vi "update-signal-values.vi"(8 "error in (no error)":errorcluster, 9 "Array":bool[](array[boolean]), 10 "TAGS":string[](array[string]), 11 "dbc in":refnum<class "dbc.lvclass">) -> (0 "error out":errorcluster, 3 "dbc out":refnum<class "dbc.lvclass">)   [LabVIEW 2015, in "dbc.lvclass"]
uses:
  dbc.lvclass
  dbc.lvclass/dbc.ctl
  <resource>/objmgr/xnet.rc
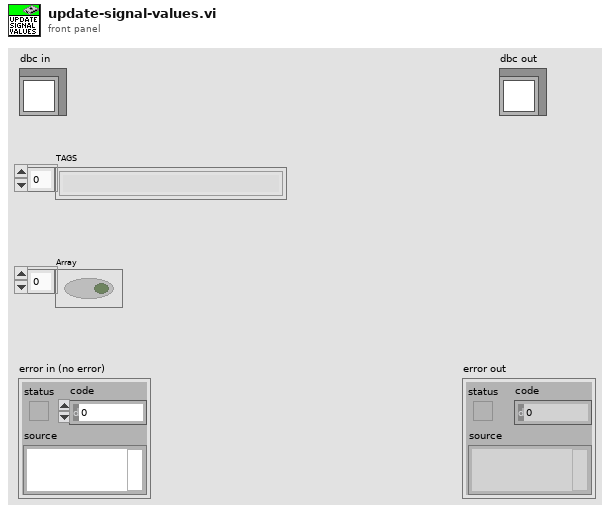
[diagram p1: front panel]
types:
  T1 = typedef "signals.result.ctl" = T2[]
  T2 = typedef "signal.result.ctl" = cluster{"Signal name":string, "payload":u8}
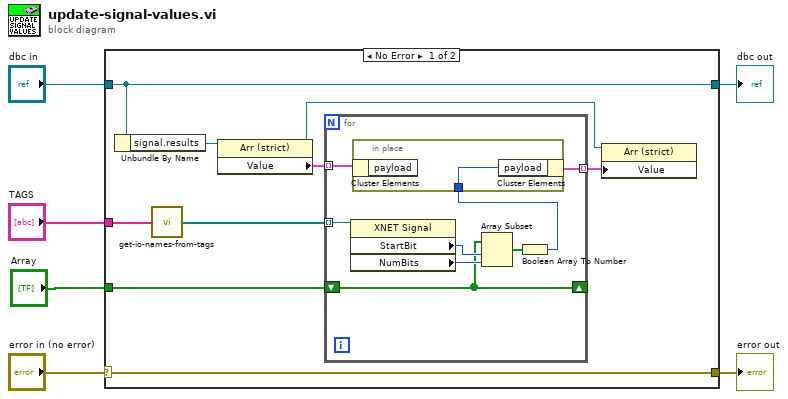
[diagram p0: block diagram]
diagram:
  n1 = case shown="No Error" "error in (no error)" {
    selector: "error in (no error)" -> [w14 w26]
    tunnel: [w14 w26] -> w5
    tunnel: [w12 w25] -> w3
    tunnel: "dbc in" -> [w12 w25]
    tunnel: "TAGS" -> [w13 _]
    tunnel: "Array" -> [w7 _]
    frame No Error {
      n2 = Unbundle By Name(w12) -> ("signal.results"=w11:refnum<vi>)
      n3 = call "get-io-names-from-tags.vi"("tags"=w13) -> ("Array"=w15:refnum<k21>[])  [unwired: 4 in]
      n4 = property class="Arr (strict)"(reference=w11) -> (reference out=w9:refnum<vi>, "Value"=w10:T1)  [unwired: 1 in, 1 out]
      n5 = for {
        tunnel: w15 -> [w23] mode=indexing
        shift-right: [w20] -> _
        shift-left: w7 -> [w20]
        tunnel: w10 -> [w19] mode=indexing
        tunnel: [w17] -> w8 mode=indexing
        n6 = property class="XNET Signal"(reference=w23) -> ("StartBit"=w21:u32, "NumBits"=w22:u32)  [unwired: 1 in, 2 out]
        n7 = Array Subset(array=w20, index=w21, length=w22) -> (w18:bool[])
        n8 = Boolean Array To Number(Boolean array=w18) -> (number=w16:u32)
        n9 = in-place {
          in-place-border: w16 -> [w24]
          n10 = in-place-cluster #1(w19) -> ()  [unwired: 1 out]
          n11 = in-place-cluster #1("payload"=w24) -> (w17:T2)
        }
      }
      n12 = property class="Arr (strict)"(reference=w9, "Value"=w8) -> ()  [unwired: 1 in, 2 out]
    }
    frame Error {
    }
  }
  "error out" <- w5
  "dbc out" <- w3
